vi "空调通讯.vi"() -> ()   [LabVIEW 2016]
uses:
  <vilib>/Plasmionique/MB Master/MB_Master/MB_Master.lvclass
  <vilib>/Plasmionique/MB Master/MB Master.lvlib
  <vilib>/Utility/config.llb/NI_LVConfig.lvlib
panel:
  out "英维克空调寄存器":u16[](array[numeric])
  in  "读取参数":bool
  in  "读取数据":bool
  in  "释放串口":bool
  in  "打开串口":bool
  out "队列中元素数量":i32
  out "元素":cluster{"命令":string}[](array[cluster])
  out "待处理插入数量":i32
  out "通讯状态":bool
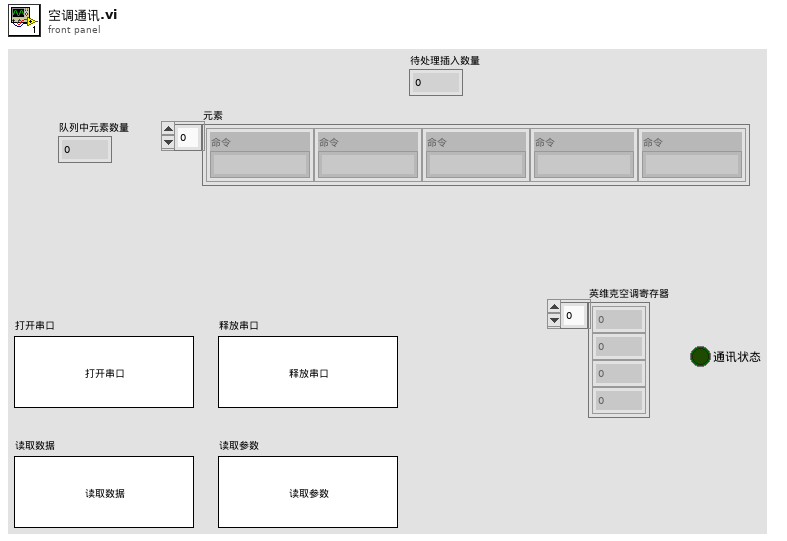
[diagram p1: front panel]
types:
  T1 = typedef "NI_LVConfig.lvlib/Config Data RefNum.ctl" = refnum<k1>
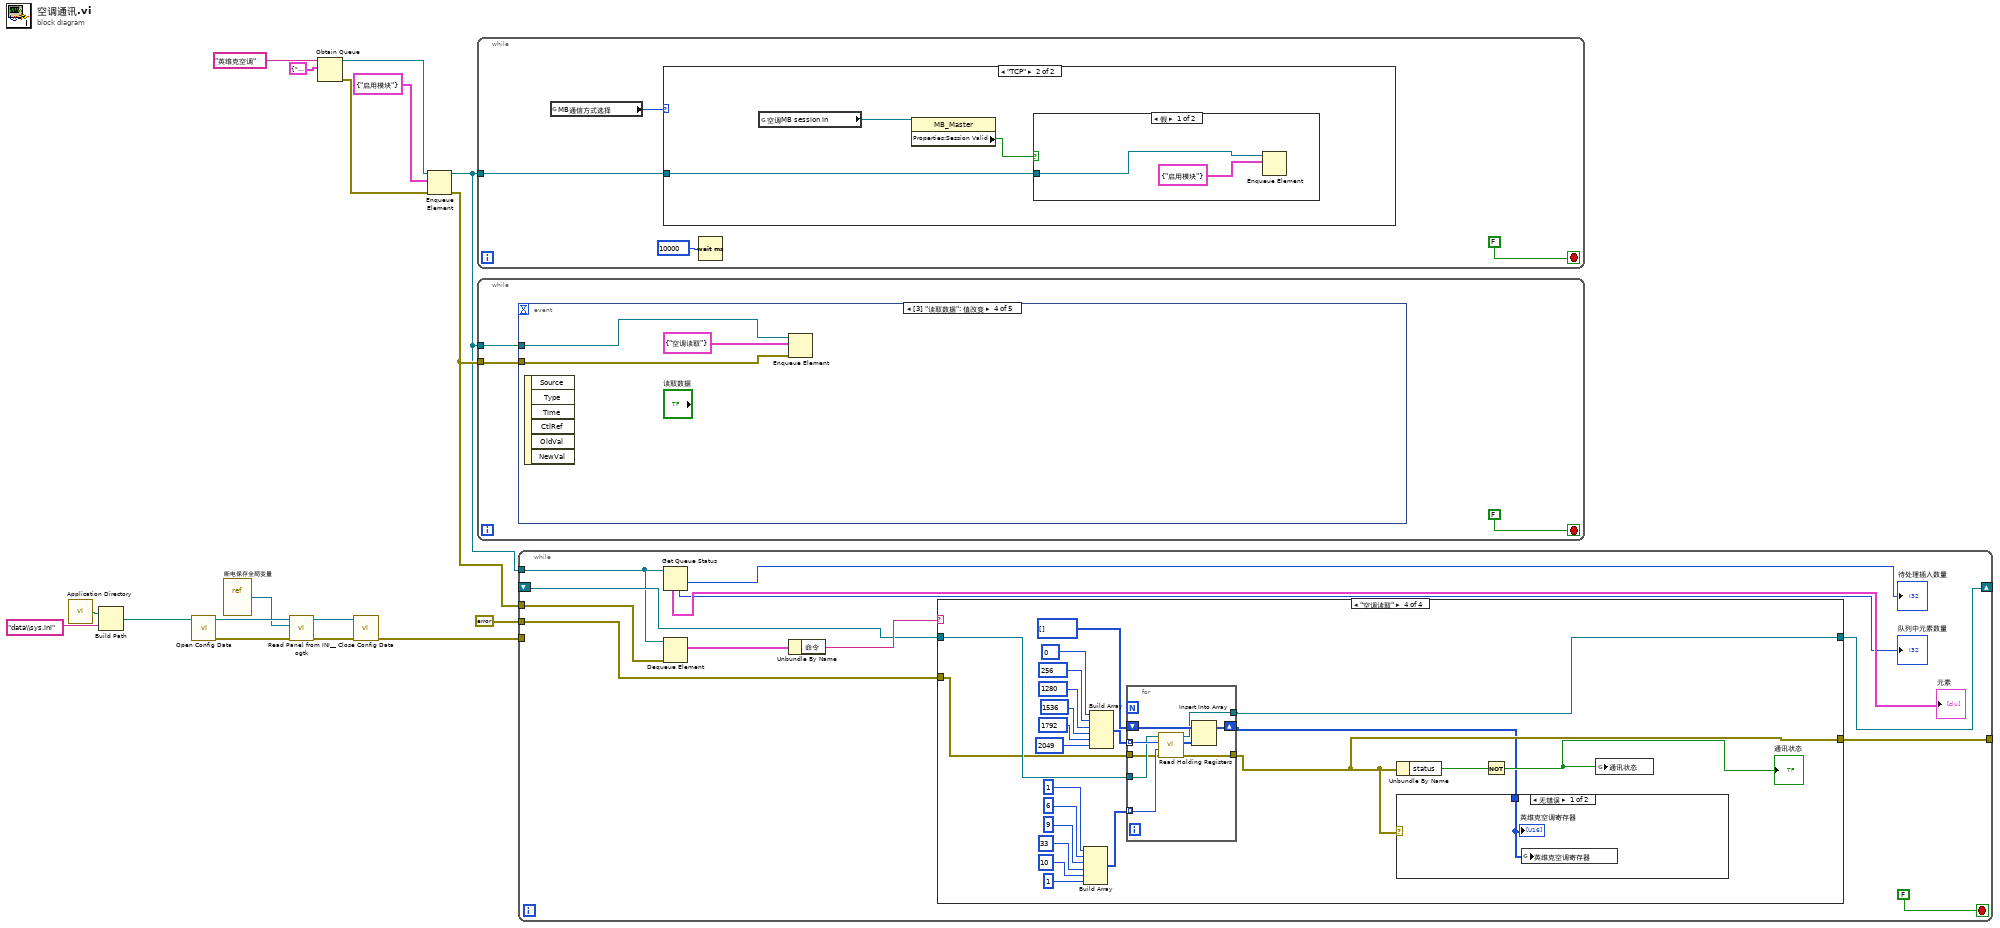
[diagram p0: block diagram]
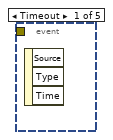
[diagram p4: hidden frame]
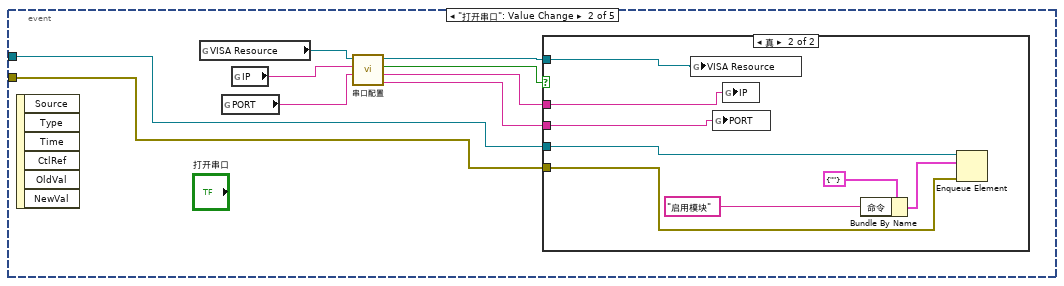
[diagram p5: hidden frame]
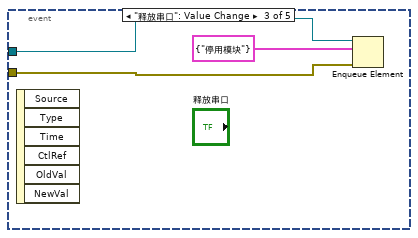
[diagram p7: hidden frame]
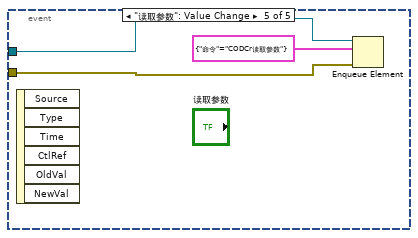
[diagram p8: hidden frame]
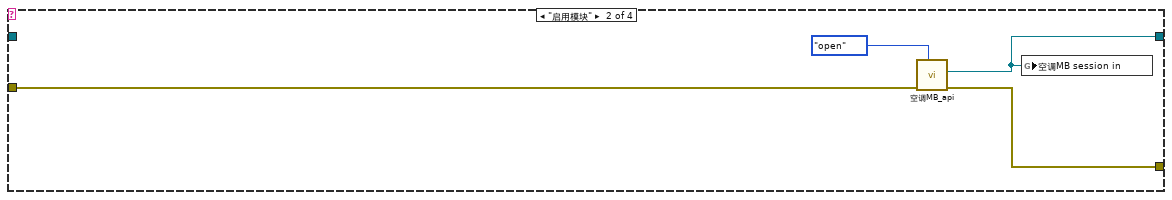
[diagram p10: hidden frame]
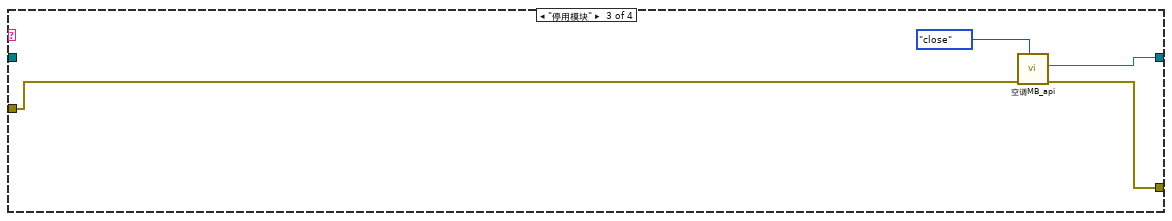
[diagram p11: hidden frame]
diagram:
  n1 = call <vilib>:"Application Directory.vi"() -> ("Application Directory"=w2:path)
  n2 = Build Path(base path=w2, name or relative path="data\\sys.ini" ("名称或相对路径")) -> (appended path=w3:path)
  n3 = call <vilib>:"Open Config Data.vi"("configuration file path"=w3) -> ("error out"=w8:errorcluster, "refnum"=w11:T1)  [unwired: 8 in, 1 out]
  n4 = vi-ref "断电保存全局变量.vi"() -> (w10:refnum<vi>)
  n5 = call <userlib>:"Read Panel from INI__ogtk.vi"("error in (no error)"=w8, "VI ref"=w10, "refnum"=w11) -> ("error out"=w7:errorcluster, "refnum out"=w9:T1)  [unwired: 7 in]
  n6 = Obtain Queue(name (unnamed)="英维克空调" ("名称（未命名）"), element data type=cluster{"命令":string} {"命令"="启用模块"} ("元素")) -> (queue out=w14:refnum<queue>, error out=w13:errorcluster)  [unwired: 3 in, 1 out]
  n7 = call <vilib>:"Close Config Data.vi"("error in (no error)"=w7, "refnum"=w9) -> ("error out"=w4:errorcluster)  [unwired: 8 in, 1 out]
  n8 = Enqueue Element(queue=w14, element=cluster{"命令":string} {"命令"="启用模块"} ("元素"), error in (no error)=w13) -> (queue out=w5:refnum<queue>, error out=w6:errorcluster)  [unwired: 1 in, 1 out]
  n9 = while {
    tunnel: w5 -> [w21]
    stop <- FALSE stop-if-true
    n10 = global read "断电保存全局变量.vi" "MB通信方式选择"() -> (w18:enum16{"串口", "TCP"})
    n11 = case shown="\"TCP\"" w18 {
      tunnel: w21 -> [_ w23]
      frame "串口", Default {
      }
      frame "TCP" {
        n12 = global read "外部交互全局变量.vi" "空调MB session in"() -> (w22:refnum<class "MB_Master.lvclass">)
        n13 = property class="MB_Master"(reference=w22) -> ("Properties:Session Valid"=w24:bool)  [unwired: 1 in, 2 out]
        n14 = case shown="假" w24 {
          tunnel: w23 -> [w26 _]
          frame False {
            n15 = Enqueue Element(queue=w26, element=cluster{"命令":string} {"命令"="启用模块"} ("元素")) -> ()  [unwired: 2 in, 3 out]
          }
          frame True {
          }
        }
      }
    }
    n16 = Wait (ms)(milliseconds to wait=u32 10000 ("等待时间（毫秒）")) -> ()  [unwired: 1 out]
  }
  n17 = while {
    tunnel: w5 -> [w28]
    tunnel: w6 -> [w27]
    stop <- FALSE stop-if-true
    n18 = event shown="[3] \"读取数据\": 值改变" {
      selector: _ -> [_ _ _ _ _]
      dyn-events: _ -> [_ _ _ _ _]
      timeout: _ -> [_ _ _ _ _]
      tunnel: w28 -> [_ w38 w49 w51 w54]
      tunnel: w27 -> [_ w37 w48 w50 w53]
      event Timeout {
        n19 = event-data() -> ()  [unwired: 1 in, 3 out]
      }
      event "打开串口": Value Change {
        n20 = event-data() -> ()  [unwired: 1 in, 6 out]
        n21 = global read "断电保存全局变量.vi" "VISA Resource"() -> (w32:refnum<visa-resource-name>)
        n22 = global read "断电保存全局变量.vi" "PORT"() -> (w30:string)
        n23 = global read "断电保存全局变量.vi" "IP"() -> (w31:string)
        n24 = call "串口配置.vi"("PORT"=w30, "IP"=w31, "请选择串口:"=w32) -> ("PORT 2"=w33:string, "IP 2"=w34:string, "确认 2"=w36:bool, "VISA资源名称 2"=w35:refnum<visa-resource-name>)  [unwired: 5 in]
        n25 = case shown="真" w36 {
          tunnel: w35 -> [_ w41]
          tunnel: w38 -> [_ w43]
          tunnel: w37 -> [_ w42]
          tunnel: w34 -> [_ w40]
          tunnel: w33 -> [_ w39]
          frame False {
          }
          frame True {
            n26 = global write "断电保存全局变量.vi" "VISA Resource"(w41) -> ()
            n27 = global write "断电保存全局变量.vi" "PORT"(w39) -> ()
            n28 = global write "断电保存全局变量.vi" "IP"(w40) -> ()
            n29 = Bundle By Name(cluster=cluster{"命令":string} {"命令"=""} ("元素"), "命令"="启用模块" ("名称（未命名）")) -> (w44:cluster{"命令":string})
            n30 = Enqueue Element(queue=w43, element=w44, error in (no error)=w42) -> ()  [unwired: 1 in, 3 out]
          }
        }
      }
      event "释放串口": Value Change {
        n31 = event-data() -> ()  [unwired: 1 in, 6 out]
        n32 = Enqueue Element(queue=w49, element=cluster{"命令":string} {"命令"="停用模块"} ("元素"), error in (no error)=w48) -> ()  [unwired: 1 in, 3 out]
      }
      event "读取数据": Value Change {
        n33 = event-data() -> ()  [unwired: 1 in, 6 out]
        n34 = Enqueue Element(queue=w51, element=cluster{"命令":string} {"命令"="空调读取"} ("元素"), error in (no error)=w50) -> ()  [unwired: 1 in, 3 out]
      }
      event "读取参数": Value Change {
        n35 = event-data() -> ()  [unwired: 1 in, 6 out]
        n36 = Enqueue Element(queue=w54, element=cluster{"命令":string} {"命令"="CODCr读取参数"} ("元素"), error in (no error)=w53) -> ()  [unwired: 1 in, 3 out]
      }
    }
  }
  n37 = while {
    tunnel: w5 -> [w59]
    tunnel: w6 -> [w66]
    tunnel: [w60] -> _
    shift-right: [w63] -> _
    shift-left: _ -> [w62]
    tunnel: errorcluster {"status"=FALSE, "code"=0, "source"=""} ("error out") -> [w61]
    tunnel: w4 -> [_]
    stop <- FALSE stop-if-true
    n38 = Get Queue Status(queue=w59) -> (# pending insert=→"待处理插入数量":i32, # elements in queue=→"队列中元素数量":i32, elements=→"元素":cluster{"命令":string}[])  [unwired: 2 in, 5 out]
    n39 = Dequeue Element(queue=w59, error in (no error)=w66) -> (element=w65:cluster{"命令":string})  [unwired: 1 in, 3 out]
    n40 = Unbundle By Name(w65) -> ("命令"=w64:string)
    n41 = case shown="\"空调读取\"" w64 {
      tunnel: [w69 w70 w74 w81] -> w63
      tunnel: [w68 w73 w75 w82] -> w60
      tunnel: w62 -> [w69 _ _ w80]
      tunnel: w61 -> [w68 w71 w76 w79]
      frame Default {
      }
      frame "启用模块" {
        n42 = call "空调MB_api.vi"("STEP"=enum16{"open", "read", "write", "close"}."open", "Error in"=w71) -> ("error out"=w73:errorcluster, "MB session out"=w70:refnum<class "MB_Master.lvclass">)  [unwired: 7 in, 1 out]
        n43 = global write "外部交互全局变量.vi" "空调MB session in"(w70) -> ()
      }
      frame "停用模块" {
        n44 = call "空调MB_api.vi"("STEP"=enum16{"open", "read", "write", "close"}."close", "Error in"=w76) -> ("error out"=w75:errorcluster, "MB session out"=w74:refnum<class "MB_Master.lvclass">)  [unwired: 7 in, 1 out]
      }
      frame "空调读取" {
        n45 = Build Array(u16 1 ("quantity"), u16 6 ("quantity"), u16 9 ("quantity"), u16 33 ("quantity"), u16 10 ("quantity"), u16 1 ("quantity")) -> (w90:u16[])
        n46 = Build Array(u16 0 ("starting address"), u16 256 ("starting address"), u16 1280 ("starting address"), u16 1536 ("starting address"), u16 1792 ("starting address"), u16 2049 ("starting address")) -> (w89:u16[])
        n47 = for {
          tunnel: w89 -> [w108] mode=indexing
          tunnel: w90 -> [w107] mode=indexing
          shift-right: [w106] -> w78
          shift-left: u16[] [] -> [w105]
          tunnel: w80 -> [w103]
          tunnel: w79 -> [w102]
          tunnel: [w101] -> w81
          tunnel: [w100] -> w82
          n48 = call <vilib>:"Read Holding Registers.vi"("error in (no error)"=w102, "quantity"=w107, "starting address"=w108, "MB session in"=w103) -> ("error out"=w100:errorcluster, "Registers"=w104:u16[], "MB session out"=w101:refnum<class "MB_Master.lvclass">)  [unwired: 5 in]
          n49 = Insert Into Array(array=w105, new element=w104) -> (w106:u16[])  [unwired: 1 in]
        }
        n50 = Unbundle By Name(w82) -> ("status"=w99:bool)
        n51 = case shown="无错误" w82 {
          tunnel: w78 -> [w109 _]
          frame No Error {
            n52 = global write "断电保存全局变量.vi" "英维克空调寄存器"(w109) -> ()
            "英维克空调寄存器" <- w109
          }
          frame Error {
          }
        }
        n53 = Not(x=w99) -> (.not. x?=w98:bool)
        "通讯状态" <- w98
        n54 = global write "断电保存全局变量.vi" "通讯状态"(w98) -> ()
      }
    }
  }
